vi "Dequeue Element.vi"(8 "error in (no error)":errorcluster, 11 "QDMH in":refnum<class "QDMH.lvclass">) -> (0 "error out":errorcluster, 1 "State":string, 2 "Data":variant, 3 "QDMH out":refnum<class "QDMH.lvclass">, 4 "Remaining":i32)   [LabVIEW 2023, in "QDMH.lvlib" / "QDMH.lvclass"]
doc: "Dequeue single element returning the individual parts of the payload\n\nReport the status of the queue buffer - this is used to monitor queue growth rate to prevent buffer overruns"
uses:
  Library/QDMH.lvclass
  Library/QDMH.lvclass/QDMH.ctl
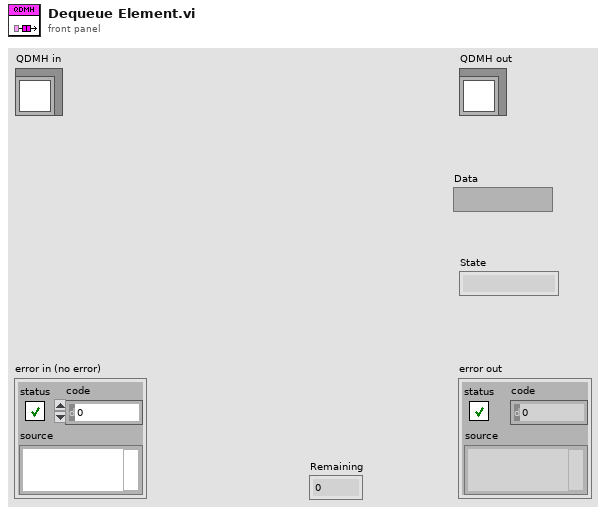
[diagram p1: front panel]
types:
  T1 = typedef "QDMH.lvlib/QDMH.lvclass/Message.ctl" = cluster{"State":string, "Data":variant}
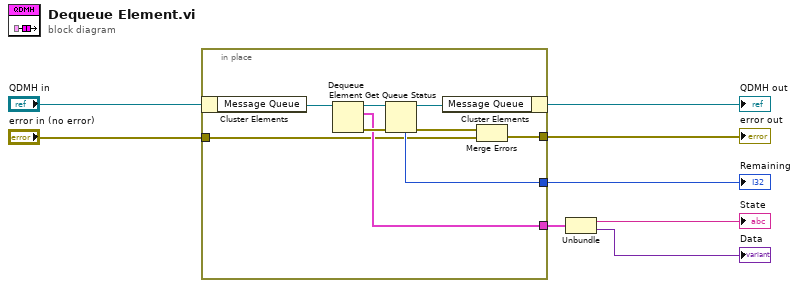
[diagram p0: block diagram]
diagram:
  n1 = in-place {
    in-place-border: [w13] -> w1
    in-place-border: [w12] -> w4
    in-place-border: "error in (no error)" -> [w9]
    in-place-border: [w10] -> w5
    n2 = in-place-cluster #1("QDMH in") -> ("Message Queue"=w17:refnum<queue>)
    n3 = Dequeue Element(queue=w17) -> (queue out=w16:refnum<queue>, element=w12:T1, error out=w14:errorcluster)  [unwired: 2 in, 1 out]
    n4 = Get Queue Status(queue=w16, error in (no error)=w14) -> (queue out=w15:refnum<queue>, error out=w11:errorcluster, # elements in queue=w13:i32)  [unwired: 1 in, 5 out]
    n5 = in-place-cluster #1("Message Queue"=w15) -> (→"QDMH out":refnum<class "QDMH.lvclass">)
    n6 = Merge Errors(w11, w9) -> (w10:errorcluster)
  }
  "error out" <- w5
  "Remaining" <- w1
  n7 = Unbundle(w4) -> ("State"=→"State":string, "Data"=→"Data":variant)
